vi "Clear Macro Data.vi"(11 "Macro":T1) -> (3 "Macro out":T1)   [LabVIEW 2023]
doc: "Clears <B>Macro</B> in preparation to create a new macro with some starting information."
uses:
  CTLs/Step Type V3.ctl
  CTLs/Step V3.ctl
  CTLs/Macro Cluster V3.ctl
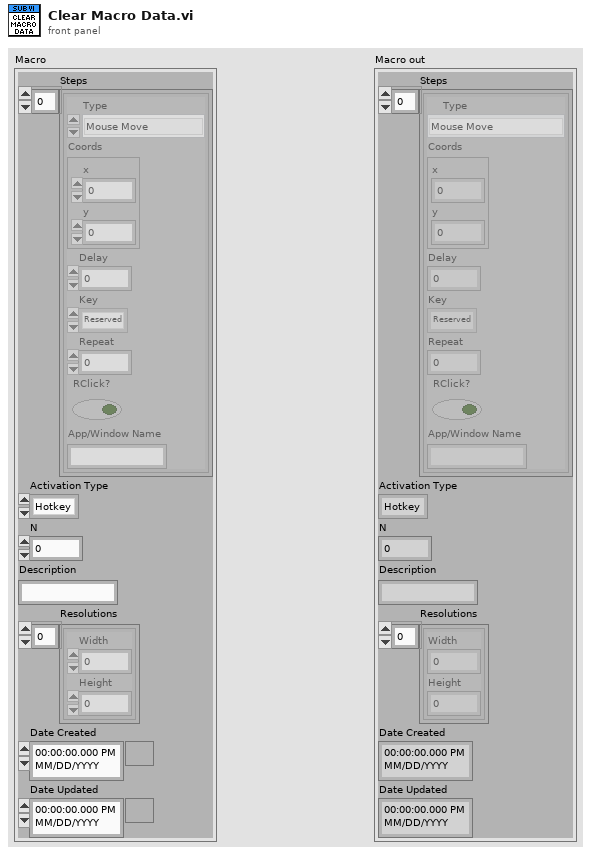
[diagram p1: front panel]
types:
  T1 = typedef "Macro Cluster V3.ctl" = cluster{"Steps":T2[], "Activation Type":enum32{"Hotkey", "Automatic"}, "N":i32, "Description":string, "Resolutions":cluster{"Width":i16, "Height":i16}[], "Date Created":timestamp, "Date Updated":timestamp}
  T2 = typedef "Step V3.ctl" = cluster{"Type":T3, "Coords":cluster{"x":i32, "y":i32}, "Delay":i32, "Key":u8, "Repeat":i32, "RClick?":bool, "App/Window Name":string}
  T3 = typedef "Step Type V3.ctl" = enum16{"Mouse Move", "Mouse Click", "Key Press", "Wait", "Mouse Down", "Mouse Up", "Key Down", "Key Up", "Run Application", "Quit Application", "Maximize Window", "Minimize Window", "Bring Window to Front", "Send Window to Back"}
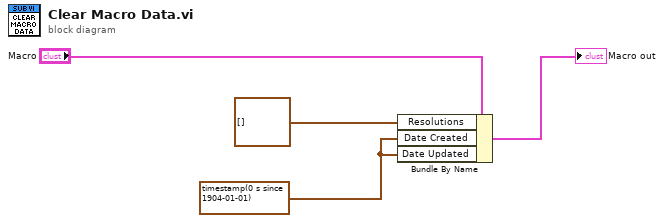
[diagram p0: block diagram]
diagram:
  w1 = timestamp(0 s since 1904-01-01) ("Date Created")
  n1 = Bundle By Name(cluster="Macro", "Resolutions"=cluster{"Width":i16, "Height":i16}[] [], "Date Created"=w1, "Date Updated"=w1) -> (→"Macro out":T1)
